vi "Write Global Locked.vi"(8 "error in (no error)":errorcluster, 10 "Global":refnum<class "System.lvclass">, 11 "DriveMotorsRight in":refnum<class "DriveMotorsRight.lvclass">) -> (0 "error out":errorcluster, 3 "DriveMotorsRight out":refnum<class "DriveMotorsRight.lvclass">)   [LabVIEW 2013]
uses:
  DriveMotorsRight.lvclass
  Robot Global Data.vi
  System/System.lvclass
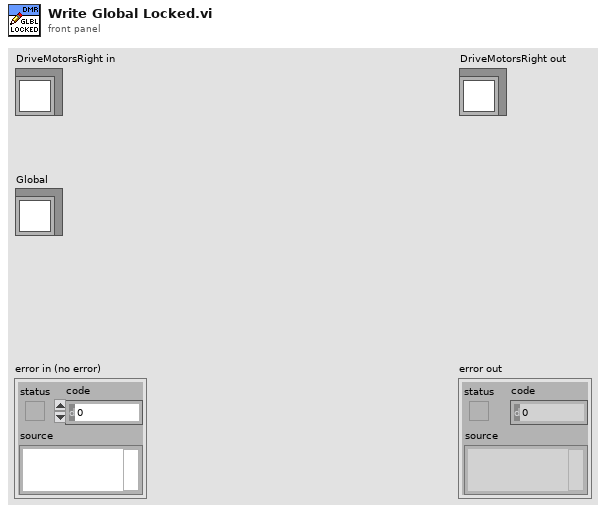
[diagram p1: front panel]
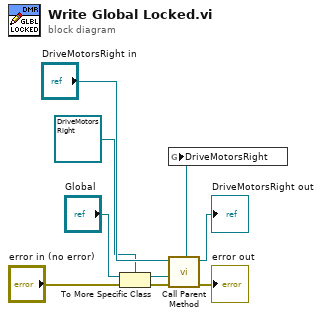
[diagram p0: block diagram]
diagram:
  n1 = To More Specific Class(target class=refnum<class "DriveMotorsRight.lvclass"> refnum ("DriveMotorsRight.lvclass"), reference="Global", error in="error in (no error)") -> (specific class reference=w3:refnum<class "DriveMotorsRight.lvclass">, error out=w1:errorcluster)
  n2 = global write "Robot Global Data.vi" "DriveMotorsRight"(w3) -> ()
  n3 = call-parent "Call Parent Method"("error in (no error)"=w1, "System in"="DriveMotorsRight in") -> ("error out"=→"error out":errorcluster, "System out"=→"DriveMotorsRight out":refnum<class "DriveMotorsRight.lvclass">)  [unwired: 8 in]
